vi "AO Config Pane.vi"(6 "_SubPanelMessages":refnum<notifier>, 9 "_myEmbeddedToFrameEvent":T7, 10 "_myEmbedded.Exit":refnum<user-event>, 11 "-Property Bundle":cluster{"Name":string, "Value":variant}[](array[cluster])) -> (1 "_Connection Informations":T1, 2 "_Scripter Input":T9)   [LabVIEW 2021]
uses:
  <vilib>/myRIO/Common/Express VI Framework/xctls/myRIO Channel List/myRIO Channel List.xctl
  <vilib>/myRIO/Common/Express VI Framework/typedefs/Config Pane to Framework Ref.ctl
  <vilib>/myRIO/Common/Express VI Framework/typedefs/Data Validate Ref.ctl
  <vilib>/myRIO/Common/Express VI Framework/typedefs/Scripter Input.ctl
  <vilib>/myRIO/Common/Express VI Framework/typedefs/WireThrough Terminal Names.ctl
  <vilib>/myRIO/Common/Express VI Framework/typedefs/Instrument Driver Method Descriptor Array.ctl
  <vilib>/myRIO/Common/Express VI Framework/typedefs/Instrument Driver Method Descriptor.ctl
  <vilib>/myRIO/Common/Express VI Framework/typedefs/Sub Panel Messages.ctl
  <vilib>/myRIO/Common/Express VI Framework/typedefs/Connection Informations.ctl
  <vilib>/myRIO/Common/Instrument Driver Framework/Utilities/typedefs/Channel Types.ctl
panel:
  in  "Selected Channel List":T2[](xcontrol)=[{"Channel Name"=0, "Channel Alias"="", "Remove Channel"=FALSE, "Index"=0}]
  in  "_Default Alias String":string
  in  "_VI Default Name (Edit and make value default)":string="Analog output (1 sample)"
  in  "Name:":string caption="Node name:"
  in  "_WireThrough Info (Edit and make value default)":T4={"WireThrough Top In"="AO Ref In", "WireThrough Bottom In"="error in (no error)", "WireThrough Top Out"="AO Ref Out", "WireThrough Bottom Out"="error out"}
  in  "_Template Array (Edit and make value default)":T5=[{"Function Name"="Smart Open", "VI Path"=path "<vilib>/myRIO/Instrument Drivers/Onboard IO/AO/vis", "Script"=TRUE, "Inputs"=[{"name"="Channel Names", "value"=variant, "Config Pane Only"=TRUE, "Build Array"=FALSE, "Bundle Cluster"=FALSE, "Show Term"=FALSE, "alias"=[], "Required Input"=FALSE}], "Outputs"=[], "VI Class"=enum."Open", "Controls Refs[]"=[], "Inline"=FALSE}, {"Function Name"="Open", "VI Path"=path "<vilib>/myRIO/Instrument Drivers/Onboard IO/AO/vis", "Script"=FALSE, "Inputs"=[{"name"="Channel Names", "value"=variant, "Config Pane Only"=TRUE, "Build Array"=FALSE, "Bundle Cluster"=FALSE, "Show Term"=FALSE, "alias"=[], "Required Input"=FALSE}], "Outputs"=[], "VI Class"=enum."Open", "Controls Refs[]"=[], "Inline"=FALSE}, {"Function Name"="Write", "VI Path"=path "<vilib>/myRIO/Instrument Drivers/Onboard IO/AO/vis", "Script"=TRUE, "Inputs"=[{"name"="Values", "value"=variant, "Config Pane Only"=FALSE, "Build Array"=TRUE, "Bundle Cluster"=FALSE, "Show Term"=TRUE, "alias"=[], "Required Input"=TRUE}], "Outputs"=[], "VI Class"=enum."Data", "Controls Refs[]"=[], "Inline"=FALSE}, {"Function Name"="Close", "VI Path"=path "<vilib>/myRIO/Instrument Drivers/Onboard IO/AO/vis", "Script"=FALSE, "Inputs"=[], "Outputs"=[], "VI Class"=enum."Close", "Controls Refs[]"=[], "Inline"=FALSE}]
  in  "_Test Close":bool
  # "User Visible Area"
  # "NOTE: Tab Order has been set\nfor this Front Panel.\n1. Name: (string control)\n2. Add Channel (button)\n3. Selected Channel List (array)\n\nAll other controls are excluded \nfrom Tabbing order\n\nTo exlude a control from context\nhelp prefix its label text with a '-'"
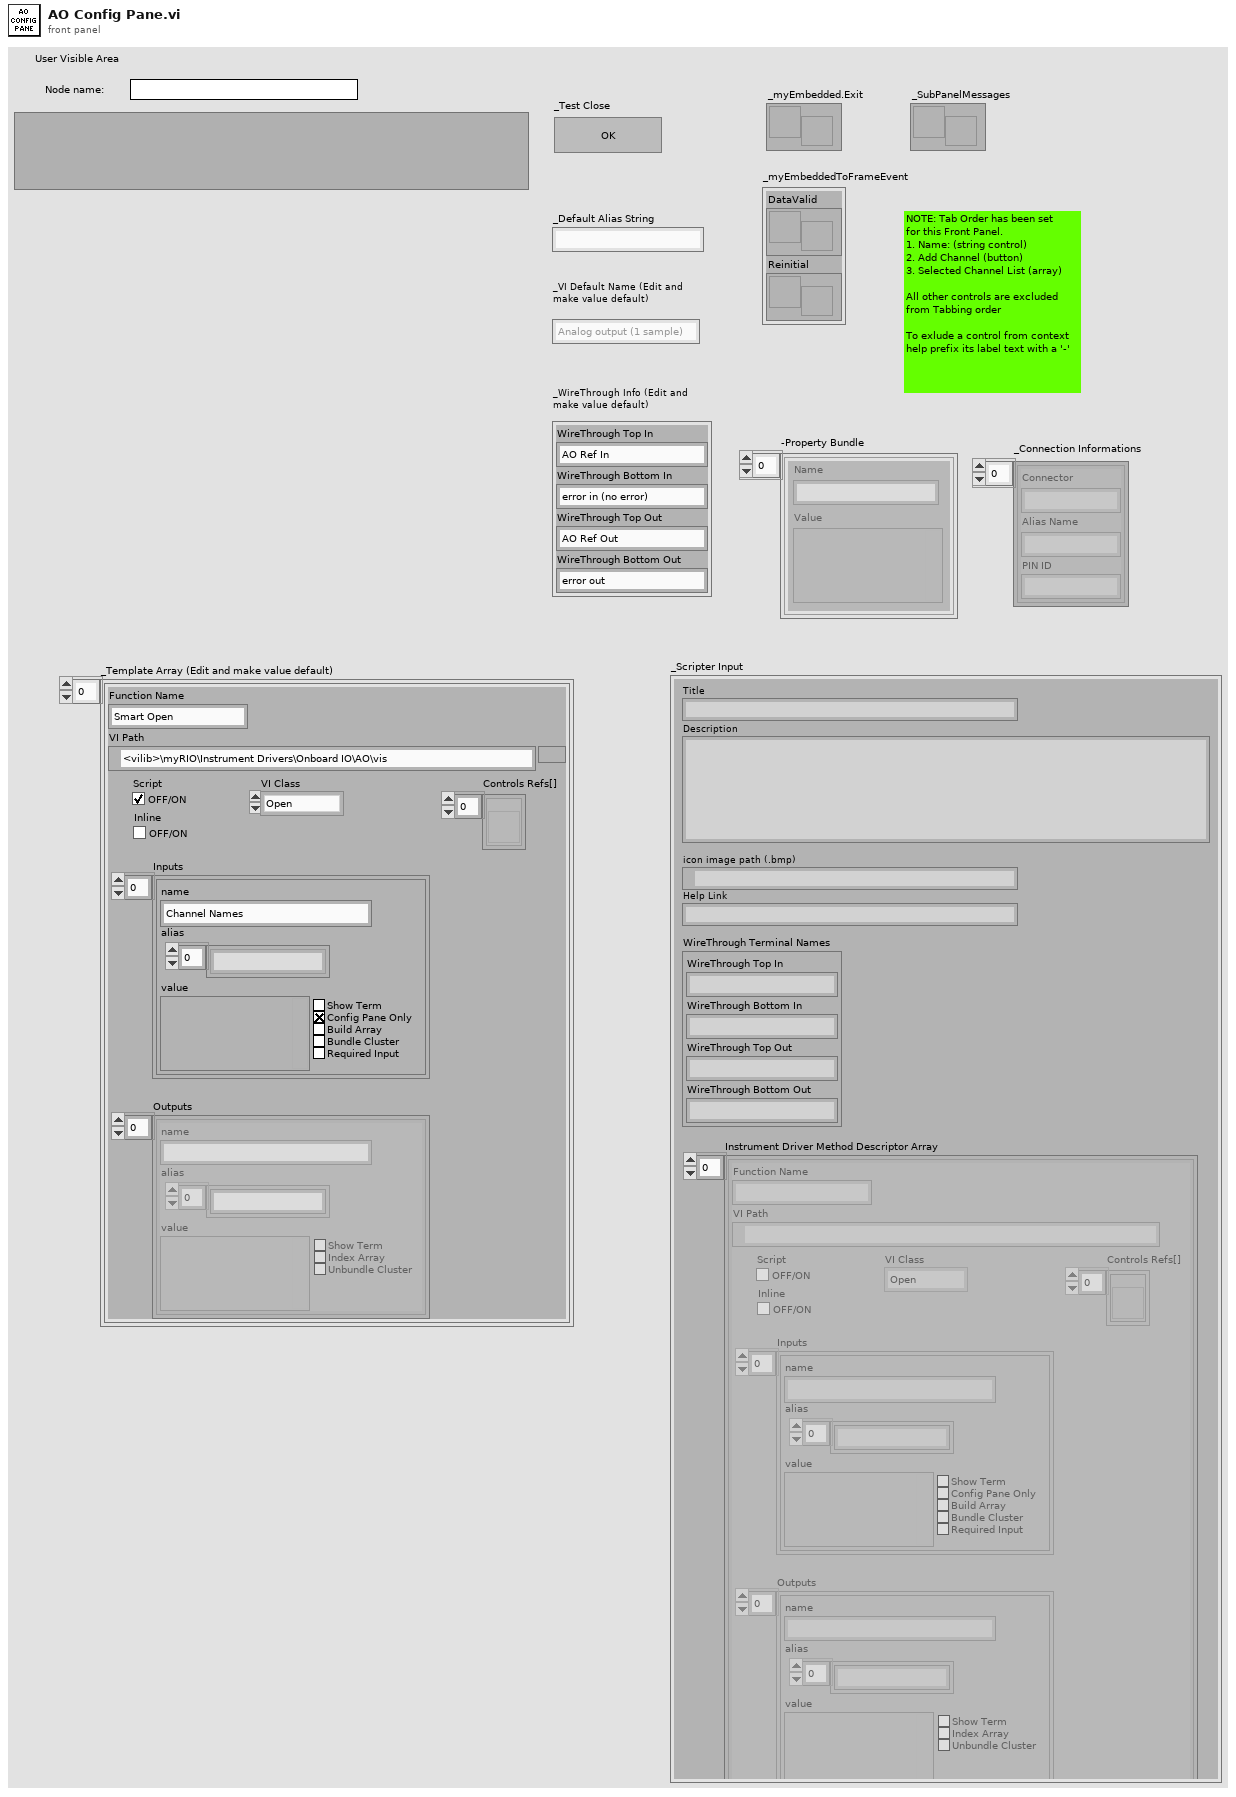
[diagram p1: front panel]
types:
  T1 = typedef "Connection Informations.ctl" = cluster{"Connector":string, "Alias Name":string, "PIN ID":string}[]
  T2 = typedef "myRIO Channel List.xctl/Channel Data.ctl" = cluster{"Channel Name":u16, "Channel Alias":string, "Remove Channel":T3, "Index":i32}
  T3 = typedef "myRIO Channel List.xctl/Remove Channel.ctl" = bool
  T4 = typedef "WireThrough Terminal Names.ctl" = cluster{"WireThrough Top In":string, "WireThrough Bottom In":string, "WireThrough Top Out":string, "WireThrough Bottom Out":string}
  T5 = typedef "Instrument Driver Method Descriptor Array.ctl" = T6[]
  T6 = typedef "Instrument Driver Method Descriptor.ctl" = cluster{"Function Name":string, "VI Path":path, "Script":bool, "Inputs":cluster{"name":string, "value":variant, "Config Pane Only":bool, "Build Array":bool, "Bundle Cluster":bool, "Show Term":bool, "alias":string[], "Required Input":bool}[], "Outputs":cluster{"name":string, "value":variant, "Show Term":bool, "Index Array":bool, "Unbundle Cluster":bool, "alias":string[]}[], "VI Class":enum16{"Open", "Configure", "Data", "Manage", "Close"}, "Controls Refs[]":refnum<vi>[], "Inline":bool}
  T7 = typedef "Config Pane to Framework Ref.ctl" = cluster{"DataValid":T8, "Reinitial":refnum<user-event>}
  T8 = typedef "Data Validate Ref.ctl" = refnum<user-event>
  T9 = typedef "Scripter Input.ctl" = cluster{"Title":string, "Description":string, "icon image path (.bmp)":path, "Help Link":string, "WireThrough Terminal Names":T4, "Instrument Driver Method Descriptor Array":T5}
  T10 = typedef "Channel Types.ctl" = enum32{"Unknown", "AI", "AO", "DIO - DI", "DIO", "DIO - DO", "I2C", "PWM", "Encoder", "SPI", "UART", "Accelerometer", "DIO - LED", "DIO - Button", "AI (N Samples)", "AudioIn (N Samples)", "AO (N Samples)", "AudioOut (N Samples)", "DI (N Samples)", "DO (N Samples)", "AI IRQ", "DI IRQ", "Timer IRQ", "RSL", "Relay", "CAN", "AI (Continuous)", "AO (Continuous)"}
  T11 = typedef "Channel Info.ctl" = cluster{"Channel Name":string, "Alias":string, "Used?":bool, "Not Support?":bool, "Property Bundle":cluster{"Name":string, "Value":variant}[]}
  T12 = typedef "Sub Panel Messages.ctl" = enum16{"Initialized"}
  T13 = cluster{"Connector":string, "Alias Name":string, "PIN ID":string}[]
  T14 = cluster{"name":string, "value":variant, "Config Pane Only":bool, "Build Array":bool, "Bundle Cluster":bool, "Show Term":bool, "alias":string[], "Required Input":bool}[]
  T15 = cluster{"name":string, "value":variant, "Config Pane Only":bool, "Build Array":bool, "Bundle Cluster":bool, "Show Term":bool, "alias":string[], "Required Input":bool}
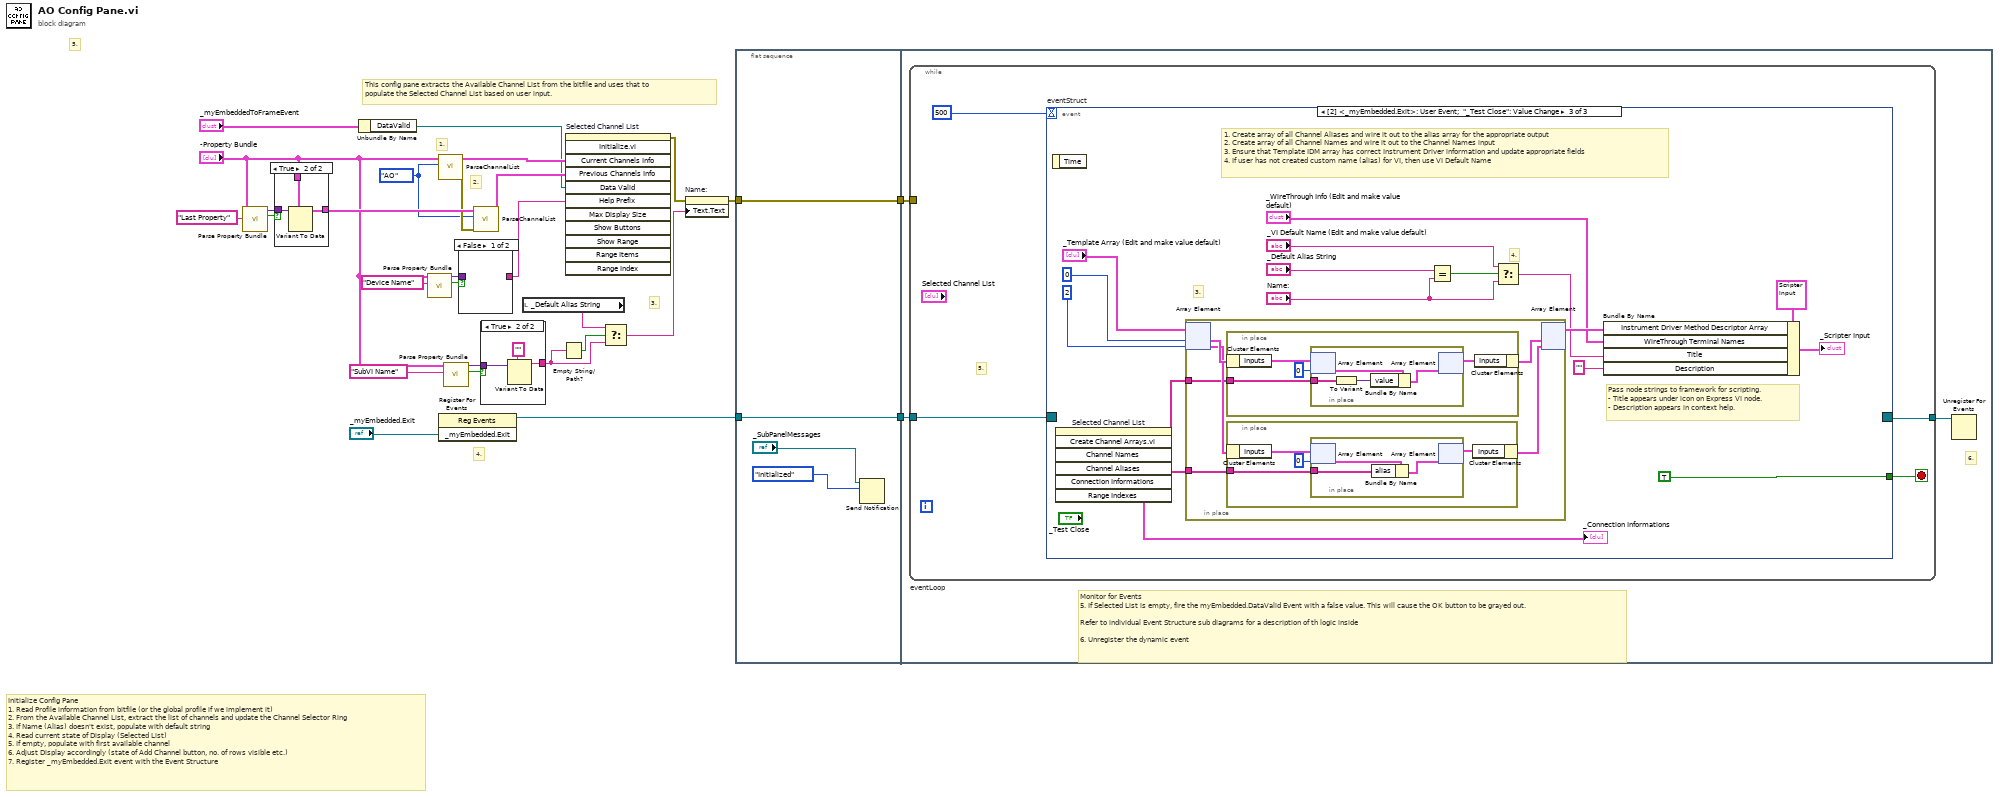
[diagram p0: block diagram]
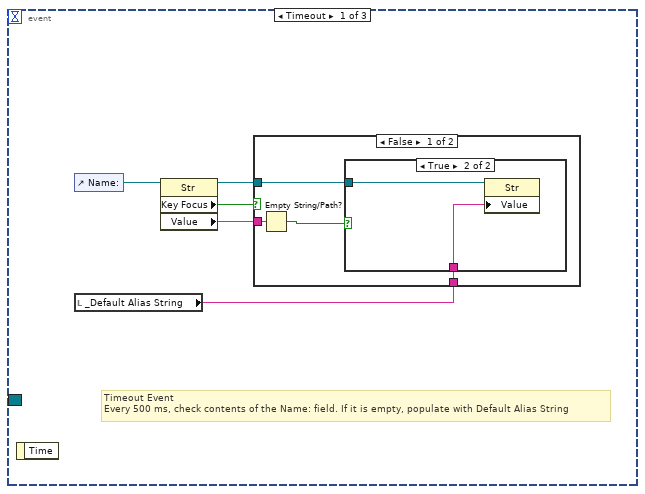
[diagram p2: hidden frame]
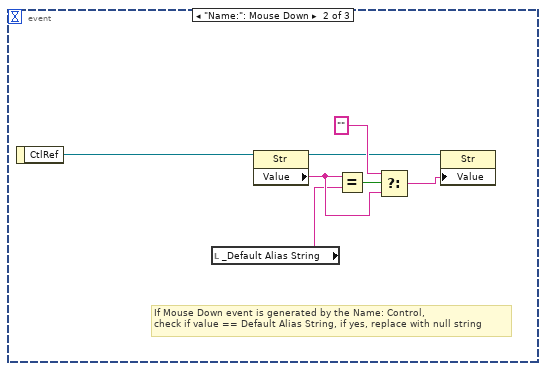
[diagram p5: hidden frame]
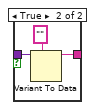
[diagram p6: hidden frame]
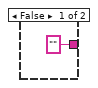
[diagram p8: hidden frame]
diagram:
  w10 = Channel_Types."AO" ("Channel to Read")
  # "2."
  # "1."
  # "This config pane extracts the Available Channel List from the bitfile and uses that to \npopulate the Selected Channel List based on user input."
  # "4."
  # "5."
  # "3."
  # "Initialize Config Pane\n1. Read Profile information from bitfile (or the global profile if we implement it)\n2. From the Available Channel List, extract the list of channels and update the Channel Selector Ring\n3. If Name (Alias) doesn't exist, populate with default string\n4. Read current state of Display (Selected List)\n5. If empty, populate with first available channel\n6. Adjust Display accordingly (state of Add Channel button, no. of rows visible etc.)\n7. Register _myEmbedded.Exit event with the Event Structure"
  n1 = call <vilib>:"Parse Property Bundle.vi"("Name"="Last Property", "Property Bundle"="-Property Bundle") -> ("Found?"=w14:bool, "Value"=w15:variant)  [unwired: 8 in]
  n2 = case shown="True" w14 {
    tunnel: w15 -> [_ w31]
    tunnel: [_ w30] -> w12
    tunnel: "-Property Bundle" -> [_ w29]
    frame False {
    }
    frame True {
      n3 = Variant To Data(type=w29, Variant=w31) -> (data=w30:cluster{"Name":string, "Value":variant}[])  [unwired: 1 in, 1 out]
    }
  }
  n4 = Unbundle By Name("_myEmbeddedToFrameEvent") -> ("DataValid"=w3:T8)
  n5 = call <vilib>:"Parse Property Bundle.vi"("Name"="Device Name", "Property Bundle"="-Property Bundle") -> ("Found?"=w8:bool, "Value"=w7:variant)  [unwired: 8 in]
  n6 = call <vilib>:"ParseChannelList.vi"("Channel to Read"=w10, "_Property Bundle"="-Property Bundle") -> ("error out"=w11:errorcluster, "Channel List Out"=w17:T11[])  [unwired: 7 in, 1 out]
  n7 = register-events("_myEmbedded.Exit") -> (reference out=w28:refnum<event-registration>)  [unwired: 2 in, 1 out]
  n8 = call <vilib>:"Parse Property Bundle.vi"("Name"="SubVI Name", "Property Bundle"="-Property Bundle") -> ("Found?"=w22:bool, "Value"=w21:variant)  [unwired: 8 in]
  n9 = case shown="False" w8 {
    tunnel: w7 -> [_ w34]
    tunnel: [_ w32] -> w6
    frame False {
    }
    frame True {
      n10 = Variant To Data(type="", Variant=w34) -> (data=w32:string)  [unwired: 1 in, 1 out]
    }
  }
  n11 = call <vilib>:"ParseChannelList.vi"("error in (no error)"=w11, "Channel to Read"=w10, "_Property Bundle"=w12) -> ("Channel List Out"=w9:T11[])  [unwired: 6 in, 2 out]
  n12 = case shown="True" w22 {
    tunnel: w21 -> [_ w38]
    tunnel: ["" ("Name") w36] -> w20
    frame False {
    }
    frame True {
      n13 = Variant To Data(type="" ("Name"), Variant=w38) -> (data=w36:string)  [unwired: 1 in, 1 out]
    }
  }
  n14 = local read "_Default Alias String"() -> (w19:string)
  n15 = Empty String/Path?(string/path=w20) -> (empty?=w26:bool)
  n16 = invoke on="Selected Channel List" class="myRIO Channel List (strict)" method="Initialize.vi"("Current Channels Info"=w17, "Previous Channels Info"=w9, "Data Valid"=w3, "Help Prefix"=w6) -> (error out=w18:errorcluster)  [unwired: 8 in, 11 out]
  n17 = Select(t=w19, s=w26, f=w20) -> (s? t:f=w25:string)
  n18 = property on="Name:" class="Str"(error in=w18, "Text.Text"=w25) -> (error out=w24:errorcluster)  [unwired: 1 in, 1 out]
  n19 = flat-sequence {
    tunnel: w24 -> [w41]
    tunnel: w28 -> [w42]
    tunnel: [w42] -> w2
    tunnel: [w41] -> w1
    tunnel: w2 -> [w45]
    tunnel: w1 -> [w43]
    frame #0 {
      n20 = Send Notification(notification=Sub_Panel_Messages."Initialized", notifier="_SubPanelMessages") -> ()  [unwired: 1 in, 2 out]
    }
    frame #1 {
      # "6."
      # "Monitor for Events\n5. If Selected List is empty, fire the myEmbedded.DataValid Event with a false value. This will cause the OK button to be grayed out.\n\nRefer to individual Event Structure sub diagrams for a description of th logic inside\n\n6. Unregister the dynamic event"
      n21 = while "eventLoop" {
        tunnel: w45 -> [w48]
        tunnel: [w47] -> w44
        tunnel: w43 -> [_]
        stop <- w49 stop-if-true
        # "5."
        n22 = event "eventStruct" shown="[2] <_myEmbedded.Exit>: User Event;  \"_Test Close\": Value Change" {
          selector: w48 -> [_ _ _]
          dyn-events: [_ _ _] -> w47
          timeout: 500 -> [_ _ _]
          tunnel: [_ _ TRUE ("_Test Close")] -> w49
          event Timeout {
            # "Timeout Event\nEvery 500 ms, check contents of the Name: field. If it is empty, populate with Default Alias String"
            n23 = event-data() -> ()  [unwired: 1 in, 1 out]
            n24 = control-ref of="Name:"() -> (w52:refnum<vi>)
            n25 = local read "_Default Alias String"() -> (w50:string)
            n26 = property on="Property Node" class="Str"(reference=w52) -> (reference out=w51:refnum<vi>, "Key Focus"=w53:bool, "Value"=w54:string)  [unwired: 1 in, 1 out]
            n27 = case shown="False" w53 {
              tunnel: w54 -> [w58 _]
              tunnel: w51 -> [w56 _]
              tunnel: w50 -> [w55 _]
              frame False {
                n28 = Empty String/Path?(string/path=w58) -> (empty?=w57:bool)
                n29 = case shown="True" w57 {
                  tunnel: w56 -> [_ w60]
                  tunnel: w55 -> [_ w59]
                  frame False {
                  }
                  frame True {
                    n30 = property on="Property Node" class="Str"(reference=w60, "Value"=w59) -> ()  [unwired: 1 in, 2 out]
                  }
                }
              }
              frame True {
              }
            }
          }
          event "Name:": Mouse Down {
            # "If Mouse Down event is generated by the Name: Control,\ncheck if value == Default Alias String, if yes, replace with null string"
            n31 = event-data() -> ("CtlRef"=w67:refnum<vi>)  [unwired: 1 in]
            n32 = local read "_Default Alias String"() -> (w61:string)
            n33 = property class="Str"(reference=w67) -> (reference out=w63:refnum<vi>, "Value"=w62:string)  [unwired: 1 in, 1 out]
            n34 = Equal?(x=w62, y=w61) -> (x = y?=w66:bool)
            n35 = Select(t="", s=w66, f=w62) -> (s? t:f=w64:string)
            n36 = property class="Str"(reference=w63, "Value"=w64) -> ()  [unwired: 1 in, 2 out]
          }
          event User Event; "_Test Close": Value Change {
            # "1. Create array of all Channel Aliases and wire it out to the alias array for the appropriate output\n2. Create array of all Channel Names and wire it out to the Channel Names input\n3. Ensure that Template IDM array has correct Instrument Driver information and update appropriate fields\n4. If user has not created custom name (alias) for VI, then use VI Default Name"
            # "4."
            # "3."
            # "Pass node strings to framework for scripting.\n- Title appears under icon on Express VI node.\n- Description appears in context help."
            n37 = event-data() -> ()  [unwired: 1 in, 1 out]
            n38 = invoke on="Selected Channel List" class="myRIO Channel List (strict)" method="Create Channel Arrays.vi"() -> ("Channel Names"=w70:string[], "Channel Aliases"=w69:string[], "Connection Informations"=→"_Connection Informations":T13)  [unwired: 7 in, 4 out]
            n39 = in-place {
              in-place-border: w70 -> [w86]
              in-place-border: w69 -> [w85]
              n40 = in-place-array #1("_Template Array (Edit and make value default)", 0, 2) -> (w90:T6, w88:T6)
              n41 = in-place {
                in-place-border: w86 -> [w100]
                n42 = in-place-cluster #2(w90) -> ("Inputs"=w101:T14)
                n43 = in-place {
                  in-place-border: w100 -> [w102]
                  n44 = in-place-array #3(w101, 0) -> (w105:T15)
                  n45 = To Variant(anything=w102) -> (Variant=w103:variant)
                  n46 = Bundle By Name(cluster=w105, "value"=w103) -> (w104:T15)
                  n47 = in-place-array #3(w104) -> (w99:T14)  [unwired: 1 out]
                }
                n48 = in-place-cluster #2("Inputs"=w99) -> (w89:T6)
              }
              n49 = in-place {
                in-place-border: w85 -> [w93]
                n50 = in-place-cluster #4(w88) -> ("Inputs"=w94:T14)
                n51 = in-place {
                  in-place-border: w93 -> [w95]
                  n52 = in-place-array #5(w94, 0) -> (w97:T15)
                  n53 = Bundle By Name(cluster=w97, "alias"=w95) -> (w96:T15)
                  n54 = in-place-array #5(w96) -> (w92:T14)  [unwired: 1 out]
                }
                n55 = in-place-cluster #4("Inputs"=w92) -> (w87:T6)
              }
              n56 = in-place-array #1(w89, w87) -> (w82:T5)  [unwired: 2 out]
            }
            n57 = Equal?(x="_Default Alias String", y="Name:") -> (x = y?=w74:bool)
            n58 = Select(t="_VI Default Name (Edit and make value default)", s=w74, f="Name:") -> (s? t:f=w72:string)
            n59 = Bundle By Name(cluster=T9 {"Title"="", "Description"="", "icon image path (.bmp)"=path "", "Help Link"="", "WireThrough Terminal Names"={"WireThrough Top In"="", "WireThrough Bottom In"="", "WireThrough Top Out"="", "WireThrough Bottom Out"=""}, "Instrument Driver Method Descriptor Array"=[]} ("Scripter Input"), "Instrument Driver Method Descriptor Array"=w82, "WireThrough Terminal Names"="_WireThrough Info (Edit and make value default)", "Title"=w72, "Description"="" ("Title")) -> (→"_Scripter Input":T9)
          }
        }
      }
      n60 = Unregister For Events(event registration refnum=w44) -> ()  [unwired: 1 in, 1 out]
    }
  }
